vi "CustomGaussianKernel1.vi"() -> (2 "array":dbl[][](array[numeric]))   [LabVIEW 2022 SP3]
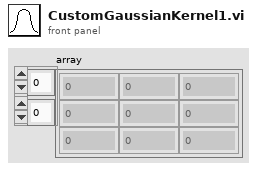
[diagram p1: front panel]
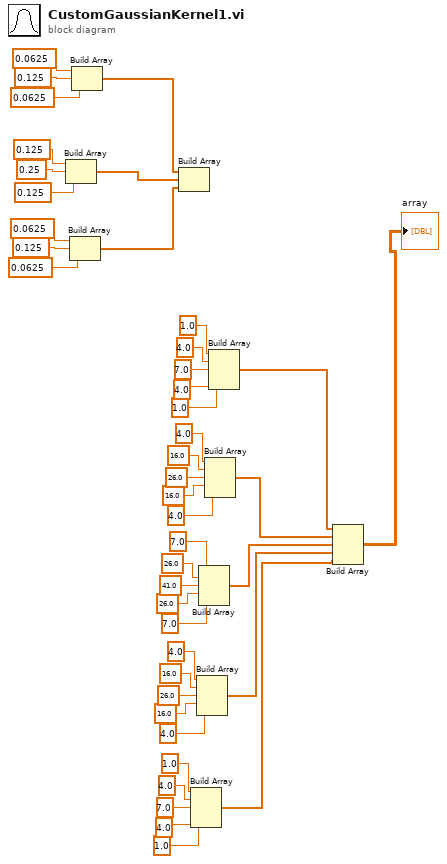
[diagram p0: block diagram]
diagram:
  n1 = Build Array(0.125 ("element"), 0.25 ("element"), 0.125 ("element")) -> (w42:dbl[])
  n2 = Build Array(0.0625 ("element"), 0.125 ("element"), 0.0625 ("element")) -> (w32:dbl[])
  n3 = Build Array(0.0625 ("element"), 0.125 ("element"), 0.0625 ("element")) -> (w43:dbl[])
  n4 = Build Array(w43, w42, w32) -> ()  [unwired: 1 out]
  n5 = Build Array(1.0 ("element"), 4.0 ("element"), 7.0 ("element"), 4.0 ("element"), 1.0 ("element")) -> (w2:dbl[])
  n6 = Build Array(4.0 ("element"), 16.0 ("element"), 26.0 ("element"), 16.0 ("element"), 4.0 ("element")) -> (w3:dbl[])
  n7 = Build Array(7.0 ("element"), 26.0 ("element"), 41.0 ("element"), 26.0 ("element"), 7.0 ("element")) -> (w4:dbl[])
  n8 = Build Array(4.0 ("element"), 16.0 ("element"), 26.0 ("element"), 16.0 ("element"), 4.0 ("element")) -> (w5:dbl[])
  n9 = Build Array(1.0 ("element"), 4.0 ("element"), 7.0 ("element"), 4.0 ("element"), 1.0 ("element")) -> (w6:dbl[])
  n10 = Build Array(w6, w5, w4, w3, w2) -> (→"array":dbl[][])
